vi "uTTA_GetLiveMeasureStatus.vi"(4 "ADC":cluster{"Offset":dbl[], "Gain":dbl[]}, 6 "PGA":cluster{"Offset":dbl[], "Gain":dbl[]}, 8 "error in":errorcluster, 9 "CalibrationMode":bool, 10 "Timeout(ms)":i32=1000, 11 "VISA Refnum in":refnum<visa-resource-name>) -> (0 "error out":errorcluster, 1 "Measurement Completed":bool, 2 "Received":string, 3 "VISA Refnum out":refnum<visa-resource-name>, 5 "MeasurementData":T2)   [LabVIEW 2021]
uses:
  CTL_uTTA_MeasurementStates.ctl
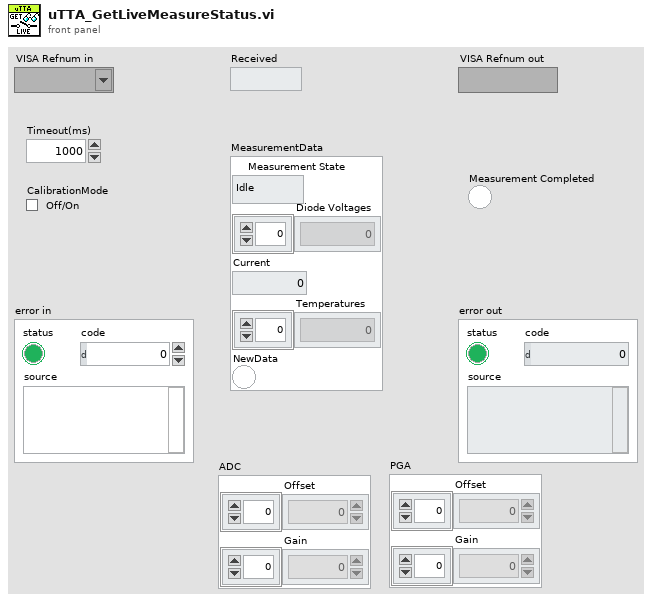
[diagram p1: front panel]
types:
  T1 = typedef "CTL_uTTA_MeasurementStates.ctl" = enum16{"Idle", "Init", "GPPowerCheck", "Preheating", "PrepHeating", "Heating", "PrepCooling", "Cooling", "Deinit", "CloseLog", "Cal_Init", "Cal_GDPowerOn", "Cal_GDPowerCheck", "Cal_Cal", "Cal_Deinit"}
  T2 = cluster{"Measurement State":T1, "Diode Voltages":dbl[], "Current":dbl, "Temperatures":dbl[], "NewData":bool}
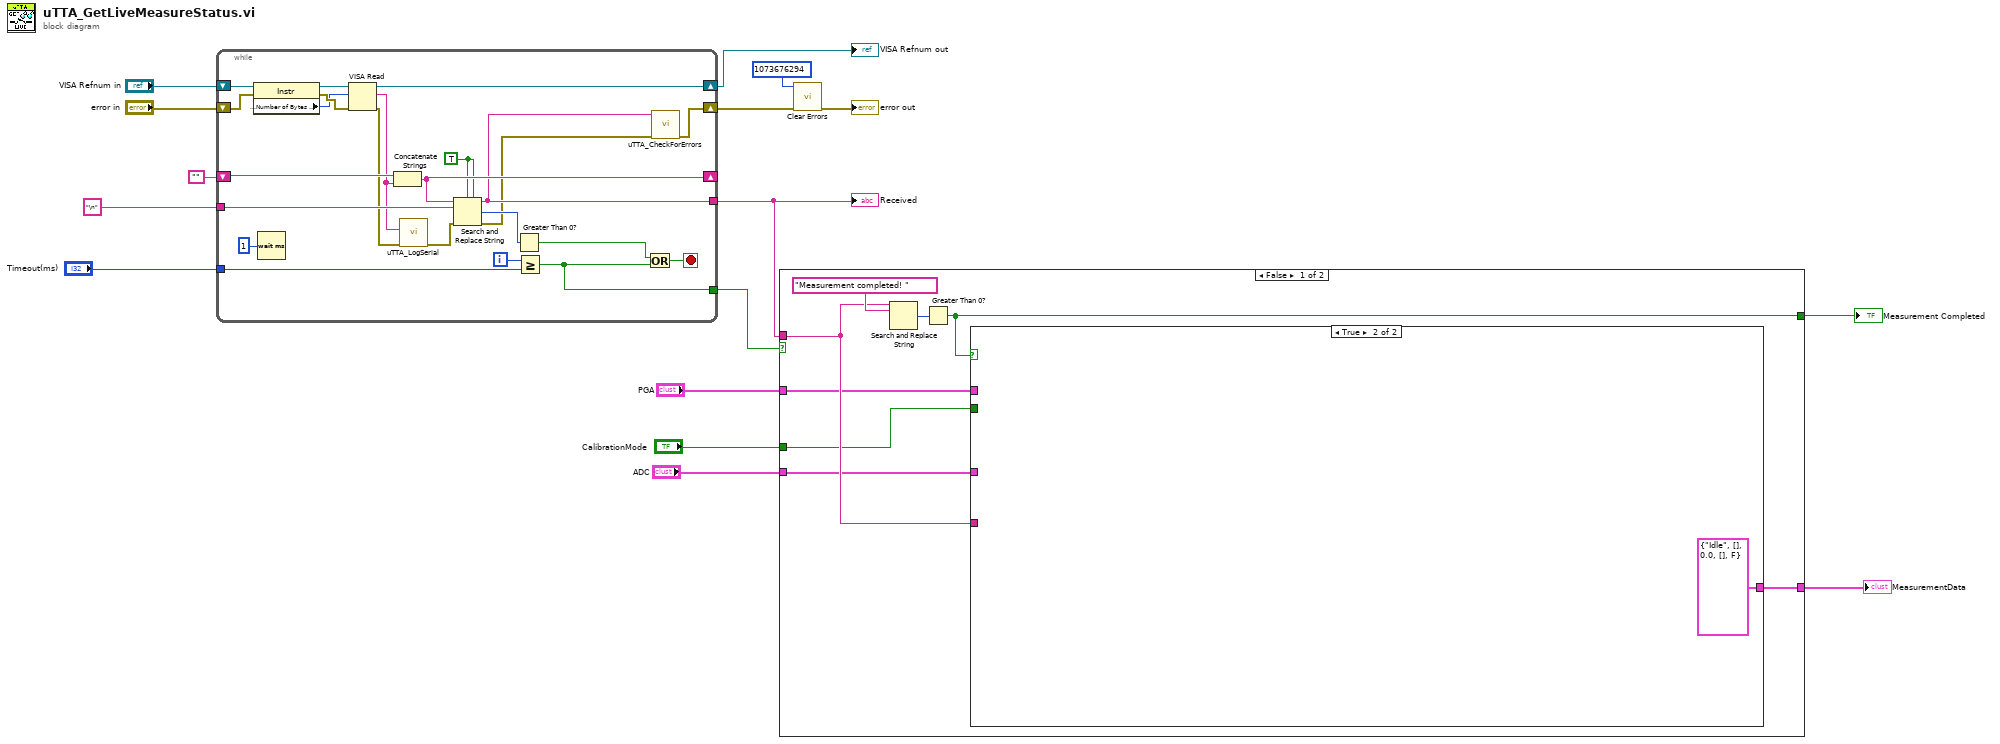
[diagram p0: block diagram]
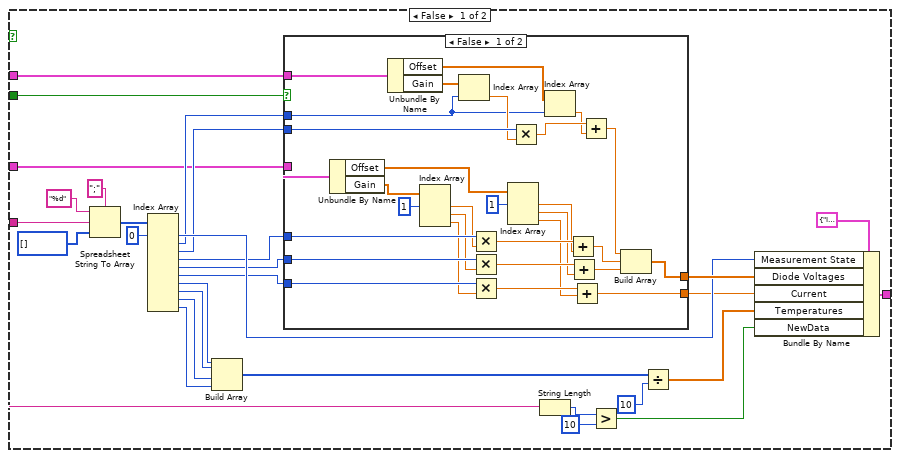
[diagram p2: hidden frame]
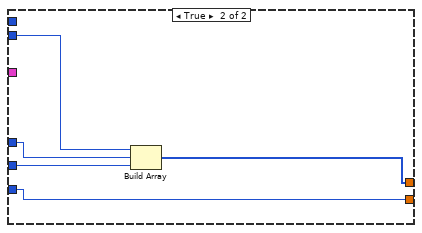
[diagram p3: hidden frame]
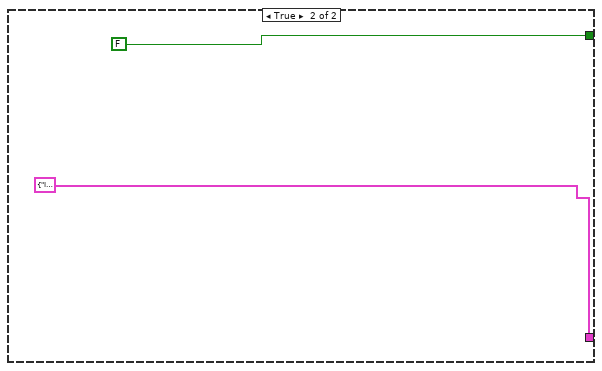
[diagram p4: hidden frame]
diagram:
  n1 = while {
    shift-right: [w33] -> _
    shift-left: "" -> [w34]
    tunnel: [w24] -> w1
    shift-right: [w22] -> w12
    shift-left: "error in" -> [w38]
    shift-right: [w30] -> w9
    shift-left: "VISA Refnum in" -> [w39]
    tunnel: "Timeout(ms)" -> [w26]
    tunnel: "\n" ("RX Termination(\\n)") -> [w25]
    tunnel: [w20] -> w7
    i -> [w27]
    stop <- w28 stop-if-true
    w21 = TRUE ("ignore case? (F)")
    n2 = property class="Instr"(reference=w39, error in=w38) -> (reference out=w37:refnum<visa-resource-name>, error out=w36:errorcluster, "Serial Settings:Number of Bytes at Serial Port"=w35:u32)
    n3 = Wait (ms)(milliseconds to wait=u32 1) -> ()  [unwired: 1 out]
    n4 = VISA Read(VISA resource name=w37, byte count=w35, error in (no error)=w36) -> (VISA resource name out=w30:refnum<visa-resource-name>, read buffer=w19:string, error out=w18:errorcluster)  [unwired: 1 out]
    n5 = Concatenate Strings(w34, w19) -> (w33:string)
    n6 = call "uTTA_LogSerial.vi"("error in"=w18, "Data_Sent"=w19) -> ("error out"=w17:errorcluster)  [unwired: 5 in]
    n7 = Search and Replace String(case sensitive?=w21, multiline?=w21, input string=w33, search string=w25, error in=w17) -> (result string=w24:string, number of replacements=w32:i32, error out=w23:errorcluster)  [unwired: 3 in, 1 out]
    n8 = Greater Than 0?(x=w32) -> (x > 0?=w29:bool)
    n9 = Greater Or Equal?(x=w27, y=w26) -> (x >= y?=w20:bool)
    n10 = Or(x=w29, y=w20) -> (x .or. y?=w28:bool)
    n11 = call "uTTA_CheckForErrors.vi"("error in"=w23, "Received"=w24) -> ("error out"=w22:errorcluster)  [unwired: 9 in]
  }
  "Received" <- w1
  "VISA Refnum out" <- w9
  n12 = case shown="False" w7 {
    tunnel: w1 -> [w44 _]
    tunnel: [w40 FALSE] -> w6
    tunnel: [w45 T2 {"Measurement State"=enum."Idle", "Diode Voltages"=[], "Current"=0.0, "Temperatures"=[], "NewData"=FALSE}] -> w5
    tunnel: "CalibrationMode" -> [w43 _]
    tunnel: "PGA" -> [w42 _]
    tunnel: "ADC" -> [w41 _]
    frame False {
      n13 = Search and Replace String(input string=w44, search string="Measurement completed! ") -> (number of replacements=w46:i32)  [unwired: 6 in, 3 out]
      n14 = Greater Than 0?(x=w46) -> (x > 0?=w40:bool)
      n15 = case shown="True" w40 {
        tunnel: [w65 T2 {"Measurement State"=enum."Idle", "Diode Voltages"=[], "Current"=0.0, "Temperatures"=[], "NewData"=FALSE}] -> w45
        tunnel: w44 -> [w52 _]
        tunnel: w43 -> [w50 _]
        tunnel: w42 -> [w49 _]
        tunnel: w41 -> [w48 _]
        frame False {
          n16 = Spreadsheet String To Array(delimiter (Tab)=";", format string="%d", spreadsheet string=w52, array type (2D Dbl)=i32[] []) -> (array=w73:i32[])
          n17 = Index Array(array=w73, index #1=0 ("index")) -> (element #1=w66:i32, element #2=w51:i32, element #3=w53:i32, element #4=w54:i32, element #5=w55:i32, element #6=w56:i32, element #7=w57:i32, element #8=w58:i32, element #9=w59:i32, element #10=w60:i32)  [unwired: 9 in]
          n18 = Build Array(w57, w58, w59, w60) -> (w69:i32[])
          n19 = case shown="False" w50 {
            tunnel: [w106 w111] -> w70
            tunnel: [w104 w107] -> w61
            tunnel: w56 -> [w97 w107]
            tunnel: w55 -> [w96 w108]
            tunnel: w54 -> [w95 w109]
            tunnel: w53 -> [w94 w110]
            tunnel: w51 -> [w91 _]
            tunnel: w49 -> [w90 _]
            tunnel: w48 -> [w87 _]
            frame False {
              n20 = Unbundle By Name(w87) -> ("Offset"=w86:dbl[], "Gain"=w80:dbl[])
              n21 = Unbundle By Name(w90) -> ("Offset"=w88:dbl[], "Gain"=w89:dbl[])
              n22 = Index Array(array=w80, index #1=1 ("index")) -> (element #1=w79:dbl, element #2=w78:dbl, element #3=w77:dbl)  [unwired: 2 in]
              n23 = Index Array(array=w89, index=w91) -> (element=w92:dbl)
              n24 = Multiply(x=w95, y=w79) -> (x*y=w101:dbl)
              n25 = Multiply(x=w96, y=w78) -> (x*y=w102:dbl)
              n26 = Multiply(x=w97, y=w77) -> (x*y=w105:dbl)
              n27 = Index Array(array=w86, index #1=1 ("index")) -> (element #1=w84:dbl, element #2=w83:dbl, element #3=w82:dbl)  [unwired: 2 in]
              n28 = Multiply(x=w94, y=w92) -> (x*y=w103:dbl)
              n29 = Index Array(array=w88, index=w91) -> (element=w93:dbl)
              n30 = Add(x=w101, y=w84) -> (x+y=w99:dbl)
              n31 = Add(x=w102, y=w83) -> (x+y=w100:dbl)
              n32 = Add(x=w105, y=w82) -> (x+y=w104:dbl)
              n33 = Add(x=w103, y=w93) -> (x+y=w98:dbl)
              n34 = Build Array(w98, w99, w100) -> (w106:dbl[])
            }
            frame True {
              n35 = Build Array(w110, w109, w108) -> (w111:i32[])
            }
          }
          n36 = String Length(string=w52) -> (length=w64:i32)
          n37 = Greater?(x=w64, y=10) -> (0:w62:bool)
          n38 = Divide(x=w69, y=10) -> (x/y=w68:dbl[])
          n39 = Bundle By Name(cluster=T2 {"Measurement State"=enum."Idle", "Diode Voltages"=[], "Current"=0.0, "Temperatures"=[], "NewData"=FALSE}, "Measurement State"=w66, "Diode Voltages"=w70, "Current"=w61, "Temperatures"=w68, "NewData"=w62) -> (w65:T2)
        }
        frame True {
        }
      }
    }
    frame True {
    }
  }
  "Measurement Completed" <- w6
  "MeasurementData" <- w5
  n40 = call <vilib>:"Clear Errors.vi"("error in (no error)"=w12, "specific error code to clear (0: all)"=1073676294) -> ("error out"=→"error out":errorcluster)  [unwired: 4 in, 1 out]
